vi "CONEX-LDS Get Positions and Power v2.vi"(11 "Connection Cluster in":T1) -> (1 "Positions":cluster{"X":dbl, "Y":dbl, "Laser Power":dbl}, 3 "Connection Cluster out":T1, 4 "Response":string)   [LabVIEW 2010]
doc: "GP - Get X, Y positions and laser power level\n\nNo inputs\n\nRead the X and Y position detected and the power detected."
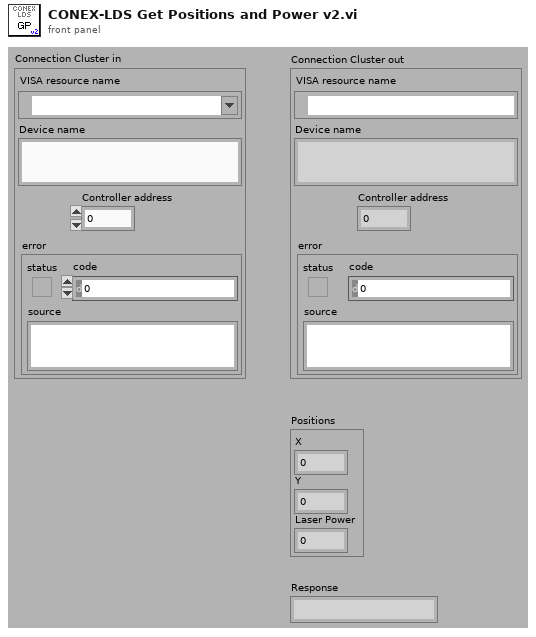
[diagram p1: front panel]
types:
  T1 = cluster{"VISA resource name":refnum<visa-resource-name>, "Device name":string, "Controller address":i32, "error":errorcluster}
  T2 = cluster{"valeur par défaut 1":dbl, "valeur par défaut 1":dbl, "valeur par défaut 1":dbl}
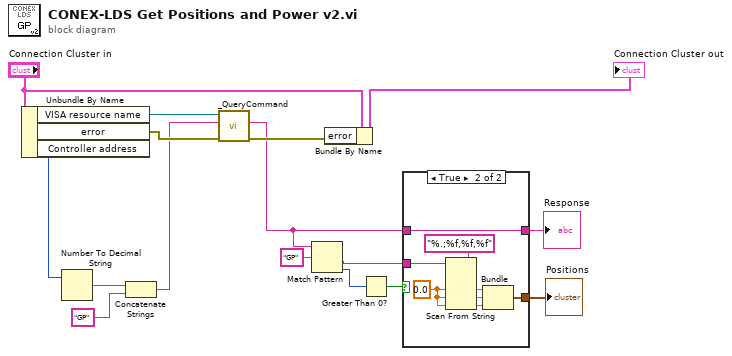
[diagram p0: block diagram]
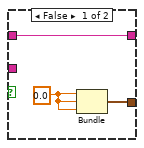
[diagram p2: hidden frame]
diagram:
  n1 = Unbundle By Name("Connection Cluster in") -> ("VISA resource name"=w8:refnum<visa-resource-name>, "error"=w7:errorcluster, "Controller address"=w3:i32)
  n2 = Number To Decimal String(number=w3) -> (decimal integer string=w16:string)  [unwired: 1 out]
  n3 = Concatenate Strings(w16, "GP" ("strCommand")) -> (w2:string)
  n4 = call <userlib>:"_QueryCommand.vi"("error in"=w7, "Command"=w2, "Instrument Channel in"=w8) -> ("error out"=w5:errorcluster, "Response"=w1:string)  [unwired: 6 in, 1 out]
  n5 = Match Pattern(string=w1, regular expression="GP" ("expression régulière")) -> (after substring=w13:string, offset past match=w12:i32)  [unwired: 3 out]
  n6 = Bundle By Name(cluster="Connection Cluster in", "error"=w5) -> (→"Connection Cluster out":T1)
  n7 = Greater Than 0?(x=w12) -> (x > 0?=w11:bool)
  n8 = case shown="True" w11 {
    tunnel: w1 -> [w17 w21]
    tunnel: w13 -> [_ w22]
    tunnel: [w17 w21] -> w10
    tunnel: [w19 w20] -> w9
    frame False {
      w18 = 0.0 ("valeur par défaut 1")
      n9 = Bundle("valeur par défaut 1"=w18, "valeur par défaut 1"=w18, "valeur par défaut 1"=w18) -> (w19:T2)  [unwired: 1 out]
    }
    frame True {
      w26 = 0.0 ("valeur par défaut 1")
      n10 = Scan From String(format string="%.;%f,%f,%f", input string=w22, default 1=w26, default 2=w26, default 3=w26) -> (output 1=w25:dbl, output 2=w24:dbl, output 3=w23:dbl)  [unwired: 2 in, 3 out]
      n11 = Bundle("valeur par défaut 1"=w25, "valeur par défaut 1"=w24, "valeur par défaut 1"=w23) -> (w20:T2)  [unwired: 1 out]
    }
  }
  "Positions" <- w9
  "Response" <- w10
